vi "CaribrationDialog.vi"() -> ()   [LabVIEW 2015]
uses:
  global.vi
panel:
  out "MSG":string
  in  "CANCEL":bool
  in  "OK":bool
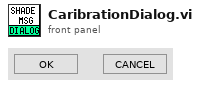
[diagram p1: front panel]
types:
  T1 = cluster{"ReturnValue":u32, "ErrorCode":u32, "error ":errorcluster}
  T2 = cluster{"return type":u32, "pErrorCode":u32, "error ":errorcluster}
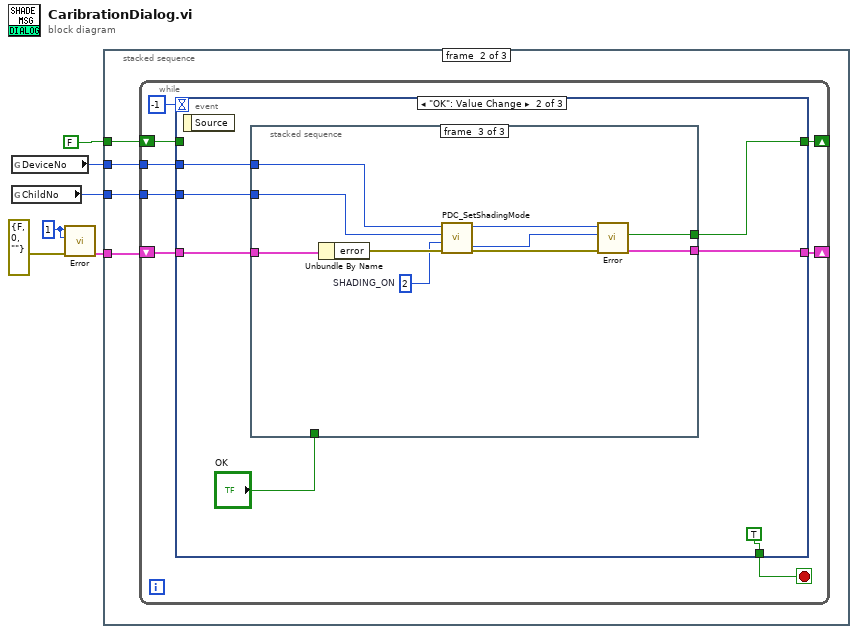
[diagram p0: block diagram]
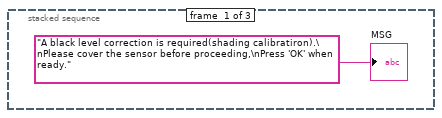
[diagram p2: hidden frame]
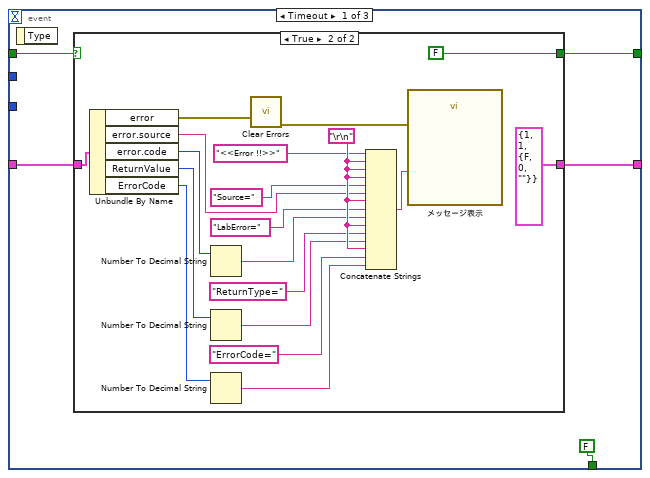
[diagram p3: hidden frame]
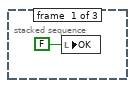
[diagram p5: hidden frame]
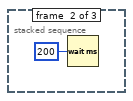
[diagram p6: hidden frame]
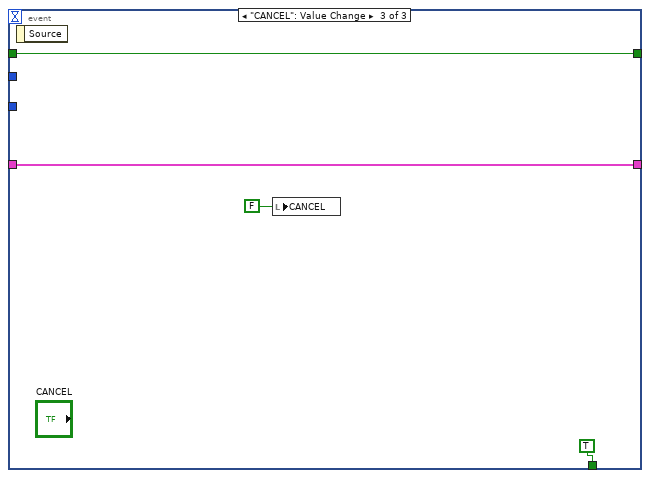
[diagram p7: hidden frame]
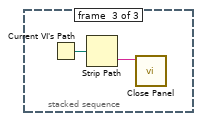
[diagram p8: hidden frame]
diagram:
  w5 = u32 1 ("return type")
  n1 = global read "global.vi" "DeviceNo"() -> (w3:u32)
  n2 = global read "global.vi" "ChildNo"() -> (w2:u32)
  n3 = call "Error.vi"("error in (no error)"=errorcluster {"status"=FALSE, "code"=0, "source"=""}, "ErrorCode"=w5, "ReturnValue"=w5) -> ("Error_Out"=w1:T1)  [unwired: 8 out]
  n4 = stacked-sequence {
    tunnel: FALSE ("Error?") -> [_ w11 _]
    tunnel: w3 -> [_ w10 _]
    tunnel: w2 -> [_ w9 _]
    tunnel: w1 -> [_ w8 _]
    frame #0 {
      "MSG" <- "A black level correction is required(shading calibratiron).\nPlease cover the sensor before proceeding,\nPress 'OK' when ready." ("MSG")
    }
    frame #1 {
      n5 = while {
        shift-right: [w16] -> _
        shift-left: w11 -> [w17]
        tunnel: w10 -> [w13]
        tunnel: w9 -> [w12]
        shift-right: [w15] -> _
        shift-left: w8 -> [w14]
        stop <- w18 stop-if-true
        n6 = event shown="[1] \"OK\": Value Change" {
          selector: _ -> [_ _ _]
          dyn-events: _ -> [_ _ _]
          timeout: -1 -> [_ _ _]
          tunnel: [FALSE TRUE TRUE] -> w18
          tunnel: w17 -> [w23 _ w67]
          tunnel: [w22 w47 w67] -> w16
          tunnel: [w21 w48 w66] -> w15
          tunnel: w14 -> [w20 w51 w66]
          tunnel: w13 -> [_ w50 _]
          tunnel: w12 -> [_ w49 _]
          event Timeout {
            n7 = event-data() -> ()  [unwired: 2 out]
            n8 = case shown="True" w23 {
              selector: w23 -> [w26 _]
              tunnel: [w26 FALSE] -> w22
              tunnel: [w25 T2 {"return type"=1, "pErrorCode"=1, "error "={"status"=FALSE, "code"=0, "source"=""}} ("Error_Out")] -> w21
              tunnel: w20 -> [w25 w27]
              frame False {
              }
              frame True {
                w44 = "\r\n"
                n9 = Unbundle By Name(w27) -> ("error"=w29:errorcluster, "error.source"=w32:string, "error.code"=w33:i32, "ReturnValue"=w36:u32, "ErrorCode"=w37:u32)
                n10 = Number To Decimal String(number=w33) -> (decimal integer string=w35:string)  [unwired: 1 out]
                n11 = Number To Decimal String(number=w36) -> (decimal integer string=w39:string)  [unwired: 1 out]
                n12 = Number To Decimal String(number=w37) -> (decimal integer string=w41:string)  [unwired: 1 out]
                n13 = call <vilib>:"Clear Errors.vi"("error in (no error)"=w29) -> ("error out"=w30:errorcluster)  [unwired: 1 in, 5 out]
                n14 = Concatenate Strings("<<Error !!>>", w44, w44, w44, "Source=", w32, w44, "LabError=", w35, w44, "ReturnType=", w39, w44, "ErrorCode=", w41) -> (w42:string)
                n15 = call "メッセージ表示"("error in (no error)"=w30, "Message"=w42) -> ()  [unwired: 1 in, 9 out]
              }
            }
          }
          event "OK": Value Change {
            n16 = event-data() -> ()  [unwired: 2 out]
            n17 = stacked-sequence {
              tunnel: w51 -> [_ _ w60]
              tunnel: w50 -> [_ _ w59]
              tunnel: w49 -> [_ _ w58]
              tunnel: [_ _ w56] -> w48
              tunnel: [_ _ w55] -> w47
              tunnel: "OK" -> [_ _ _]
              frame #0 {
                n18 = local write "OK"(FALSE ("OK")) -> ()
              }
              frame #1 {
                n19 = Wait (ms)(milliseconds to wait=u32 200 ("ミリ秒待ち時間")) -> ()  [unwired: 1 out]
              }
              frame #2 {
                w57 = u32 2  # SHADING_ON
                n20 = Unbundle By Name(w60) -> ("error"=w64:errorcluster)
                n21 = call "PDC_SetShadingMode.vi"("error in (no error)"=w64, "Mode"=w57, "ChildNo"=w58, "DeviceNo"=w59) -> ("error out"=w63:errorcluster, "ReturnValue"=w62:u32, "ErrorCode"=w61:u32)  [unwired: 5 out]
                n22 = call "Error.vi"("error in (no error)"=w63, "ErrorCode"=w61, "ReturnValue"=w62) -> ("Error_Out"=w56:T1, "Error?"=w55:bool)  [unwired: 7 out]
              }
            }
          }
          event "CANCEL": Value Change {
            n23 = event-data() -> ()  [unwired: 2 out]
            n24 = local write "CANCEL"(FALSE ("CANCEL")) -> ()
          }
        }
      }
    }
    frame #2 {
      n25 = Current VI's Path() -> (path=w69:path)
      n26 = Strip Path(path=w69) -> (name=w70:string)  [unwired: 1 out]
      n27 = call <vilib>:"Close Panel.vi"("VI name"=w70) -> ()  [unwired: 1 in, 10 out]
    }
  }
